vi "Object DAO JSON CRUD Test.vi"() -> ()   [LabVIEW 2020]
doc: "This is a Test VI for a DAO object. Here we validate CRUD Operations."
uses:
  Source Code/Object/Object.lvclass
  C:/Users/fflores/Desktop/DataBase - Copy - Copy/iOrder/iObject.lvclass
  Source Code/Object/Object.lvclass/Object.ctl
  Source Code/Object/Member Accessors/Get String.vi
  Source Code/Object/Member Accessors/Get Numeric.vi
  Source Code/Object/Member Accessors/Get Boolean.vi
  Source Code/Object/Member Accessors/Set Boolean.vi
  Source Code/Object/Member Accessors/Set Numeric.vi
  Source Code/Object/Member Accessors/Set String.vi
  Source Code/Object DAO JSON/Object DAO JSON.lvclass
  C:/Users/fflores/Desktop/DataBase - Copy - Copy/Object DAO/Object DAO.lvclass
  Source Code/Object DAO Adapter/Object DAO Adapter.lvclass
panel:
  out "Table":string[][](table)
  in  "Inputs":T1
  in  "Stop Button":bool
  in  "Delete":bool
  in  "Update":bool
  in  "Search Criteria":string
  out "Item Updated?":bool
  in  "Retrieve":bool
  in  "Create":bool
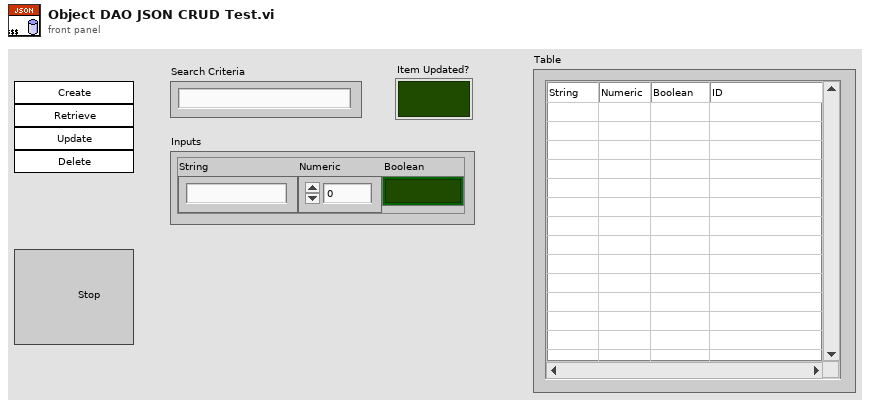
[diagram p1: front panel]
types:
  T1 = cluster{"String":string, "Numeric":dbl, "Boolean":bool}
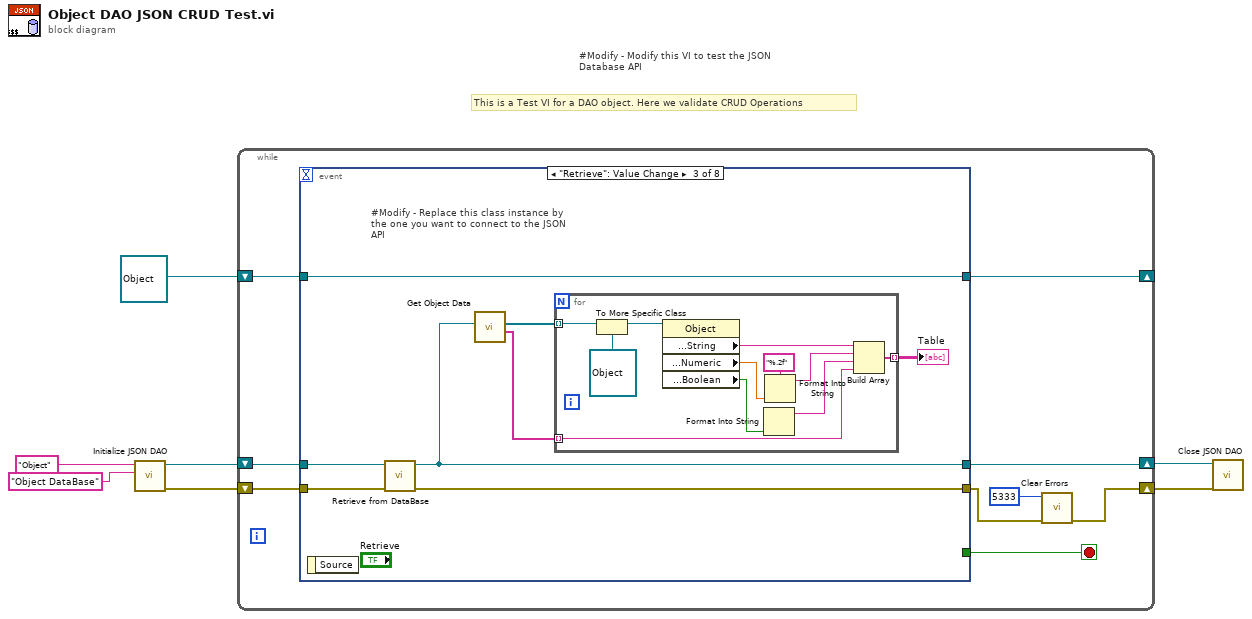
[diagram p0: block diagram]
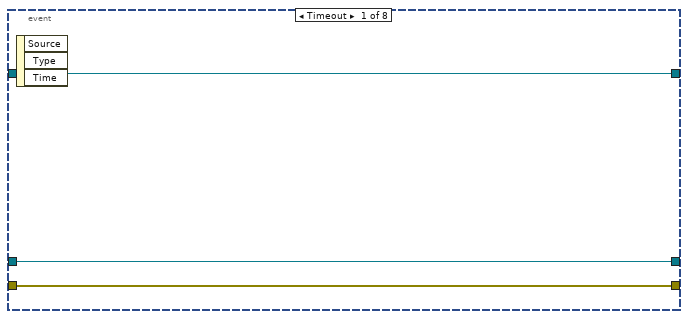
[diagram p2: hidden frame]
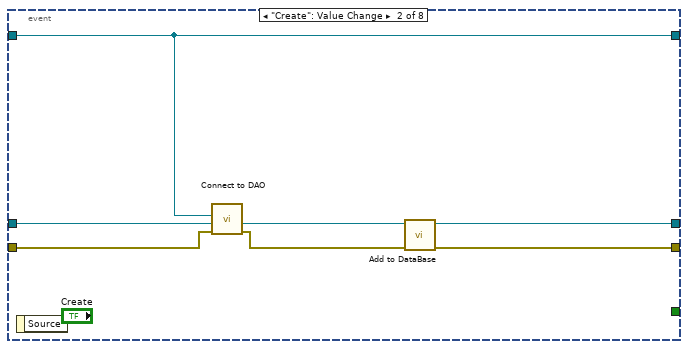
[diagram p3: hidden frame]
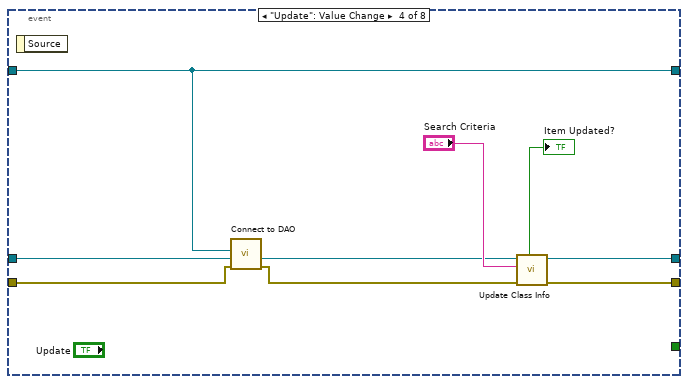
[diagram p4: hidden frame]
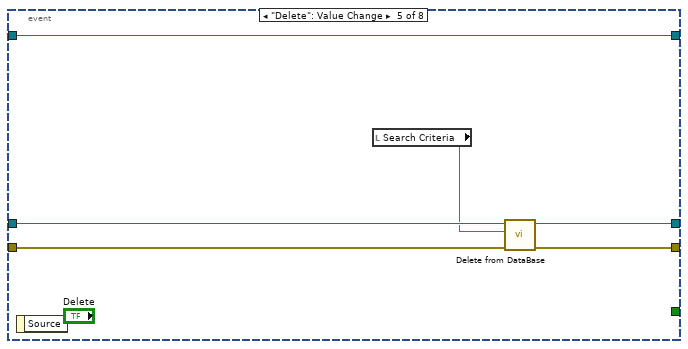
[diagram p5: hidden frame]
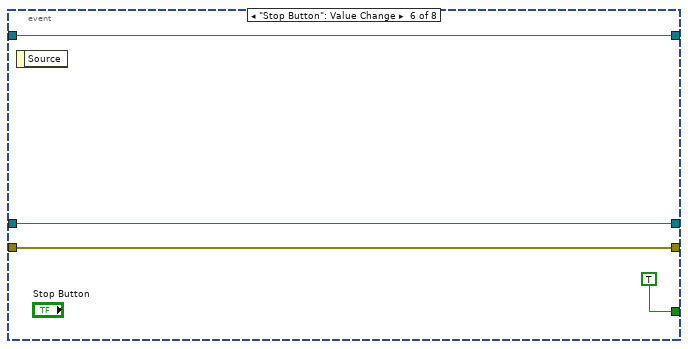
[diagram p6: hidden frame]
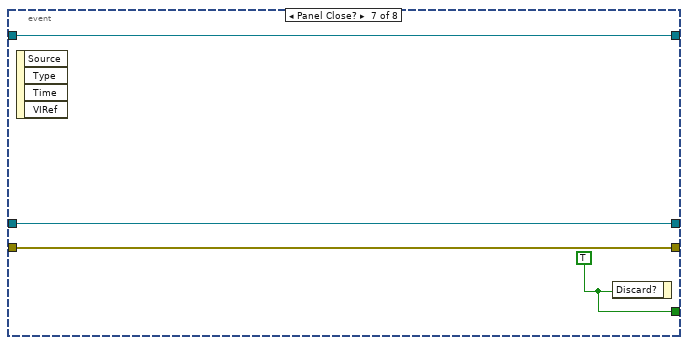
[diagram p7: hidden frame]
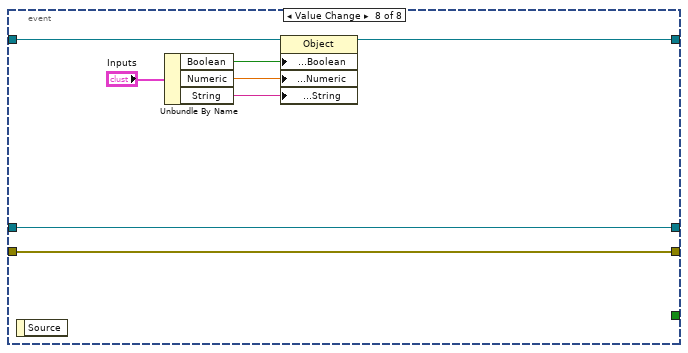
[diagram p8: hidden frame]
diagram:
  # "#Modify - Modify this VI to test the JSON Database API"
  # "This is a Test VI for a DAO object. Here we validate CRUD Operations"
  n1 = call "Initialize JSON DAO.vi"("Item Name"="Object DataBase", "DB Sufix"="Object") -> ("error out"=w6:errorcluster, "Customer DAO JSON out"=w7:refnum<class "Object DAO JSON.lvclass">)  [unwired: 8 in]
  n2 = while {
    shift-right: [w9] -> w4
    shift-left: w6 -> [w15]
    shift-right: [w13] -> w5
    shift-left: w7 -> [w16]
    shift-right: [w10] -> _
    shift-left: refnum<class "Object.lvclass"> refnum ("Object") -> [w11]
    stop <- w14 stop-if-true
    n3 = event shown="[2] \"Retrieve\": Value Change" {
      selector: _ -> [_ _ _ _ _ _ _ _]
      dyn-events: _ -> [_ _ _ _ _ _ _ _]
      timeout: _ -> [_ _ _ _ _ _ _ _]
      tunnel: w16 -> [w19 w24 w31 w49 w58 w63 w67 w76]
      tunnel: w15 -> [w18 w22 w34 w47 w60 w62 w66 w75]
      tunnel: [_ _ _ _ _ TRUE w68 _] -> w14
      tunnel: [w19 w25 w30 w53 w57 w63 w67 w76] -> w13
      tunnel: [w18 w26 w33 w54 w59 w62 w66 w75] -> w12
      tunnel: [w17 w20 w32 w50 w55 w61 w65 w73] -> w10
      tunnel: w11 -> [w17 w20 w32 w50 w55 w61 w65 w74]
      event Timeout {
        n4 = event-data() -> ()  [unwired: 1 in, 3 out]
      }
      event "Create": Value Change {
        n5 = event-data() -> ()  [unwired: 1 in, 1 out]
        n6 = call "Connect to DAO.vi"("error in (no error)"=w22, "Object DAO JSON"=w24, "iObject"=w20) -> ("error out"=w21:errorcluster, "Object DAO JSON out"=w23:refnum<class "Object DAO JSON.lvclass">)  [unwired: 7 in]
        n7 = call-dynamic "Add to DataBase.vi"("error in (no error)"=w21, "Object DAO JSON in"=w23) -> ("error out"=w26:errorcluster, "Object DAO JSON out"=w25:refnum<class "Object DAO JSON.lvclass">)  [unwired: 8 in]
      }
      event "Retrieve": Value Change {
        # "#Modify - Replace this class instance by the one you want to connect to the JSON API"
        n8 = event-data() -> ()  [unwired: 1 in, 1 out]
        n9 = call-dynamic "Retrieve from DataBase.vi"("error in (no error)"=w34, "Product DAO JSON in"=w31) -> ("error out"=w33:errorcluster, "Product DAO JSON out"=w30:refnum<class "Object DAO JSON.lvclass">)  [unwired: 8 in]
        n10 = call "Get Object Data.vi"("Object DAO"=w30) -> ("ids"=w28:string[], "Objects"=w29:refnum<class "iObject.lvclass">[])  [unwired: 8 in, 1 out]
        n11 = for {
          tunnel: w29 -> [w45] mode=indexing
          tunnel: w28 -> [w41] mode=indexing
          tunnel: [w40] -> w27 mode=indexing
          n12 = To More Specific Class(target class=refnum<class "Object.lvclass"> refnum ("Object"), reference=w45) -> (specific class reference=w36:refnum<class "Object.lvclass">)  [unwired: 1 in, 1 out]
          n13 = property class="Object"(reference=w36) -> ("Member Accessors:String"=w39:string, "Member Accessors:Numeric"=w43:dbl, "Member Accessors:Boolean"=w38:bool)  [unwired: 1 in, 2 out]
          n14 = Format Into String(w38) -> (resulting string=w37:string)  [unwired: 3 in, 1 out]
          n15 = Format Into String(format string="%.2f", w43) -> (resulting string=w42:string)  [unwired: 2 in, 1 out]
          n16 = Build Array(w39, w42, w37, w41) -> (w40:string[])
        }
        "Table" <- w27
      }
      event "Update": Value Change {
        n17 = event-data() -> ()  [unwired: 1 in, 1 out]
        n18 = call "Connect to DAO.vi"("error in (no error)"=w47, "Object DAO JSON"=w49, "iObject"=w50) -> ("error out"=w46:errorcluster, "Object DAO JSON out"=w48:refnum<class "Object DAO JSON.lvclass">)  [unwired: 7 in]
        n19 = call-dynamic "Update Class Info.vi"("error in (no error)"=w46, "Item ID"="Search Criteria", "Customer DAO JSON in"=w48) -> ("error out"=w54:errorcluster, "Item Updated?"=→"Item Updated?":bool, "Customer DAO JSON out"=w53:refnum<class "Object DAO JSON.lvclass">)  [unwired: 6 in]
      }
      event "Delete": Value Change {
        n20 = event-data() -> ()  [unwired: 1 in, 1 out]
        n21 = local read "Search Criteria"() -> (w56:string)
        n22 = call-dynamic "Delete from DataBase.vi"("error in (no error)"=w60, "Item ID"=w56, "Customer DAO JSON in"=w58) -> ("error out"=w59:errorcluster, "Customer DAO JSON out"=w57:refnum<class "Object DAO JSON.lvclass">)  [unwired: 7 in]
      }
      event "Stop Button": Value Change {
        n23 = event-data() -> ()  [unwired: 1 in, 1 out]
      }
      event Panel Close? {
        w68 = TRUE ("Discard?")
        n24 = event-data() -> ()  [unwired: 1 in, 4 out]
        n25 = event-data("Discard?"=w68) -> ()  [unwired: 1 in, 1 out]
      }
      event "Inputs.String", "Inputs.Boolean", "Inputs.Numeric": Value Change {
        n26 = event-data() -> ()  [unwired: 1 in, 1 out]
        n27 = Unbundle By Name("Inputs") -> ("Boolean"=w71:bool, "Numeric"=w70:dbl, "String"=w69:string)
        n28 = property class="Object"(reference=w74, "Member Accessors:Boolean"=w71, "Member Accessors:Numeric"=w70, "Member Accessors:String"=w69) -> (reference out=w73:refnum<class "Object.lvclass">)  [unwired: 1 in, 1 out]
      }
    }
    n29 = call <vilib>:"Clear Errors.vi"("error in (no error)"=w12, "specific error code to clear (0: all)"=5333) -> ("error out"=w9:errorcluster)  [unwired: 4 in, 1 out]
  }
  n30 = call "Close JSON DAO.vi"("error in (no error)"=w4, "Customer DAO JSON in"=w5) -> ()  [unwired: 9 in, 1 out]
